vi "onSubscribe.vi"(6 "timeout (0ms : no ack)":i32, 8 "error in (no error)":errorcluster, 10 "SUBSCRIBE":refnum<class "SUBSCRIBE.lvclass">, 11 "Client in":refnum<class "Client.lvclass">) -> (0 "error out":errorcluster, 2 "SUBACK":refnum<class "SUBACK.lvclass">, 3 "Client out":refnum<class "Client.lvclass">)   [LabVIEW 2013, in "MQTT Server.lvlib" / "Client.lvclass"]
uses:
  Client.lvclass
  Control Packets/SUBSCRIBE/SUBSCRIBE.lvclass
  Control Packets/SUBACK/SUBACK.lvclass
  MQTT_Base/MQTT_Base.lvclass
  Client.lvclass/Client.ctl
  Server/Session/Session.lvclass
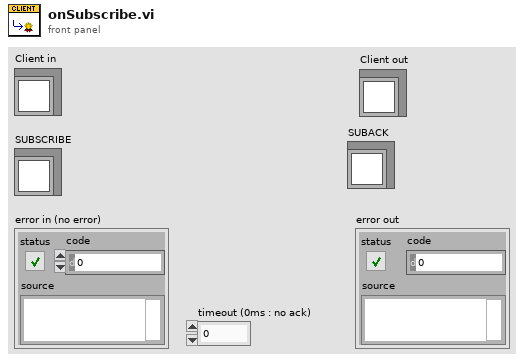
[diagram p1: front panel]
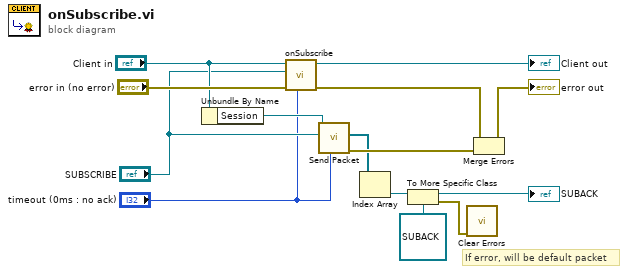
[diagram p0: block diagram]
diagram:
  # "If error, will be default packet"
  n1 = Unbundle By Name("Client in") -> ("Session"=w10:refnum<class "Session.lvclass">)
  n2 = call-parent "onSubscribe.vi"("timeout (0ms : no ack)"="timeout (0ms : no ack)", "error in (no error)"="error in (no error)", "SUBSCRIBE"="SUBSCRIBE", "MQTT_Base in"="Client in") -> ("error out"=w8:errorcluster, "MQTT_Base out"=→"Client out":refnum<class "Client.lvclass">)  [unwired: 5 in, 1 out]
  n3 = call "Send Packet.vi"("timeout (0ms : no ack)"="timeout (0ms : no ack)", "Packet"="SUBSCRIBE", "Session in"=w10) -> ("error out"=w9:errorcluster, "Response"=w5:refnum<class "ControlPacket.lvclass">[])  [unwired: 5 in, 2 out]
  n4 = Index Array(array=w5) -> (element=w4:refnum<class "ControlPacket.lvclass">)  [unwired: 1 in]
  n5 = To More Specific Class(target class=refnum<class "SUBACK.lvclass"> refnum ("SUBACK.lvclass"), reference=w4) -> (specific class reference=→"SUBACK":refnum<class "SUBACK.lvclass">, error out=w1:errorcluster)  [unwired: 1 in]
  n6 = call <vilib>:"Clear Errors.vi"("error in (no error)"=w1) -> ()  [unwired: 6 in, 1 out]
  n7 = Merge Errors(w8, w9) -> (→"error out":errorcluster)
